vi "Convert I16 to SGL.vi"(9 "Input Valid":bool, 10 "Input":i16) -> (1 "Output Valid":bool, 2 "Output":fxp<+,32,32>)   [LabVIEW 2012]
uses:
  <vilib>/rvi/IPIntegrationNode/IPINode_Utilities/niFpgaIPINodeSimCore.vi
  <vilib>/rvi/FXPMathLib/basic elements/FxpDiscreteDelay/XNode/nifxpmath_DiscreteDelay.xnode
  <vilib>/rvi/XilinxIP/XIPIN_XNode/niFpgaXIPIN.xnode
  <userlib>/FPGA Library/Code Development/SGL/Convert I16 to SGL/I16toSGL/I16toSGL_001E118E4F0B52D245E7DA9B0D265918.dll
  <vilib>/rvi/IPIntegrationNode/IPINode_Xnode/niFpgaIPINode.xnode
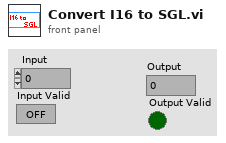
[diagram p1: front panel]
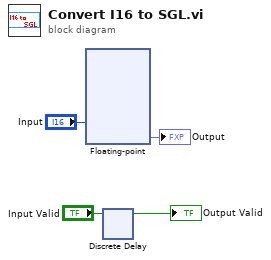
[diagram p0: block diagram]
diagram:
  n1 = xnode ("Floating-point")("a"="Input") -> ("result"=→"Output":fxp<+,32,32>)
  n2 = xnode "Discrete Delay"("D"="Input Valid") -> ("Q"=→"Output Valid":bool)
